vi "Set Data.vi"(8 "error in (no error)":errorcluster, 9 "Check Data":bool[](array[boolean]), 10 "Cell Data":string[][](array[string]), 11 "MCListbox with Checkboxes in":refnum<class "MCListbox with Checkboxes.lvclass">) -> (0 "error out":errorcluster, 3 "MCListbox with Checkboxes out":refnum<class "MCListbox with Checkboxes.lvclass">)   [LabVIEW 2016, in "MCListbox with Checkboxes.lvclass"]
uses:
  MCListbox with Checkboxes.lvclass
  MCListbox with Checkboxes.lvclass/MCListbox with Checkboxes.ctl
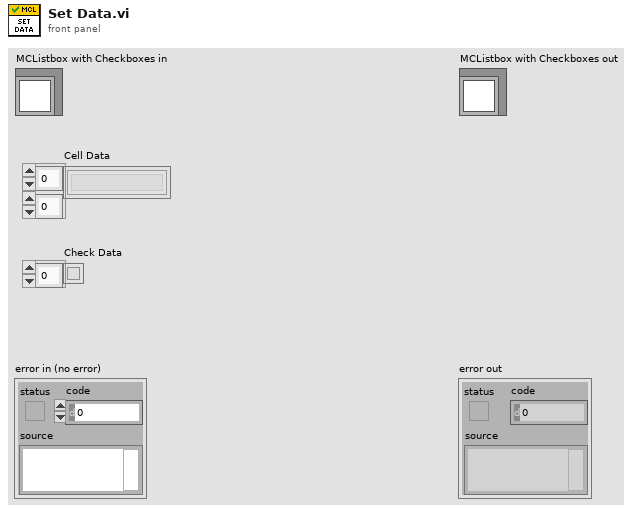
[diagram p1: front panel]
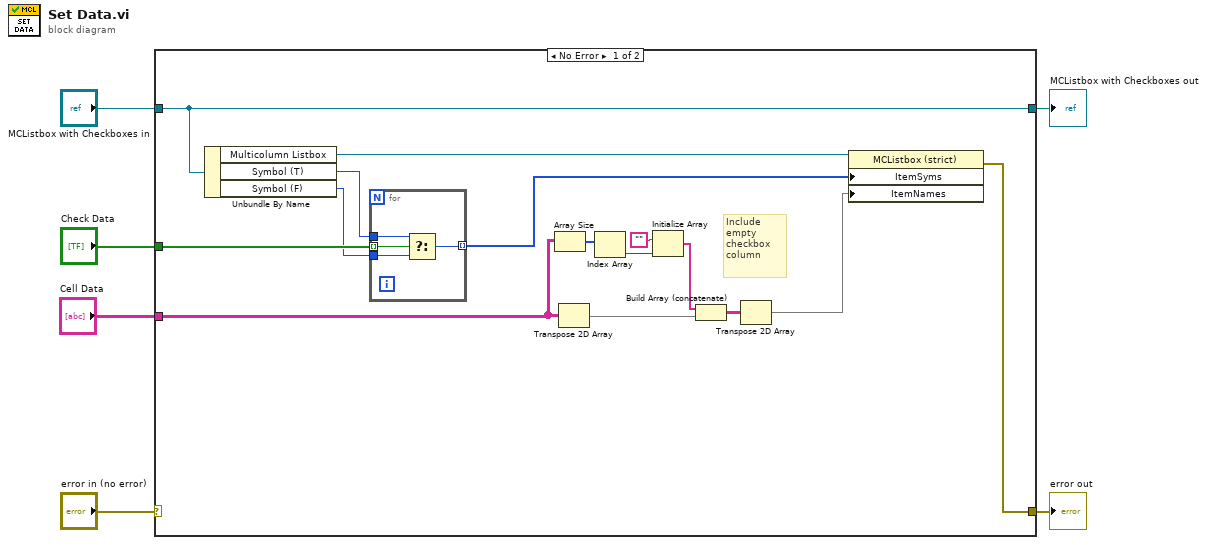
[diagram p0: block diagram]
diagram:
  n1 = case shown="No Error" "error in (no error)" {
    selector: "error in (no error)" -> [_ w27]
    tunnel: [w7 w27] -> w5
    tunnel: [w14 w26] -> w3
    tunnel: "MCListbox with Checkboxes in" -> [w14 w26]
    tunnel: "Cell Data" -> [w15 _]
    tunnel: "Check Data" -> [w12 _]
    frame No Error {
      # "Include empty checkbox column"
      n2 = Unbundle By Name(w14) -> ("Multicolumn Listbox"=w13:refnum<vi>, "Symbol (T)"=w10:i32, "Symbol (F)"=w9:i32)
      n3 = for {
        tunnel: w12 -> [w25] mode=indexing
        tunnel: w10 -> [w24]
        tunnel: w9 -> [w23]
        tunnel: [w22] -> w8 mode=indexing
        n4 = Select(t=w24, s=w25, f=w23) -> (s? t:f=w22:i32)
      }
      n5 = Array Size(array=w15) -> (size(s)=w16:i32[])
      n6 = Transpose 2D Array(2D array=w15) -> (transposed array=w20:string[][])
      n7 = Index Array(array=w16) -> (element=w18:i32)  [unwired: 1 in]
      n8 = Initialize Array("", w18) -> (w19:string[])
      n9 = Build Array (concatenate)(w19, w20) -> (w21:string[][])
      n10 = Transpose 2D Array(2D array=w21) -> (transposed array=w11:string[][])
      n11 = property class="MCListbox (strict)"(reference=w13, "ItemSyms"=w8, "ItemNames"=w11) -> (error out=w7:errorcluster)  [unwired: 1 in, 1 out]
    }
    frame Error {
    }
  }
  "error out" <- w5
  "MCListbox with Checkboxes out" <- w3
